vi "Hi_Tec_Control.vi"(0 "Carrier 1 Voltage":dbl(knob) min=0.0 max=5.0 scale=0.0..5.0 scale format="%.1f", 1 "Carrier 2 Voltage":dbl(knob) min=0.0 max=5.0 scale=0.0..5.0 scale format="%.1f", 2 "Trace Voltage":dbl(knob) min=0.0 max=5.0 scale=0.0..5.0 scale format="%.1f", 4 "Client Name":string) -> ()   [LabVIEW 2010]
uses:
  Anemometry/Anemometry Sub Vis/Controls/In_Range.ctl
  ADAM Client/Sub VIs/ADAM Controls/Update_scan_value.ctl
panel:
  out "Second stage":dbl[][](graph)
  out "First stage":dbl[][](graph)
  out "Increasing trace":bool
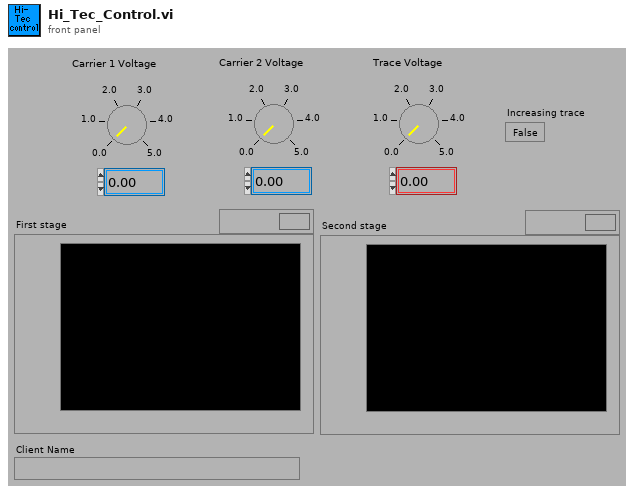
[diagram p1: front panel]
types:
  T1 = typedef "In_Range.ctl" = enum16{"%", "±", "% & ±"}
  T2 = typedef "Update_scan_value.ctl" = cluster{"Channel Name":string, "New Value":dbl}
  T3 = enum16{"Append to Global", "Read Global then Clear"}
  T4 = typedef "Ch_description_ADAM.ctl" = cluster{"Ch Name":string, "Type":T5, "Function":T6, "Ch State":T7, "Calibration type":T8, "A":dbl, "B":dbl, "C":dbl, "D":dbl, "Comments":string, "Address":T9, "String":string, "Duty":u16}
  T5 = typedef "Module_type_ADAM.ctl" = enum16{"4011", "4012", "4013", "4014", "4016", "4017", "4018", "4021", "4050", "4052", "4053", "4060", "4080", "5000", "5017", "5018", "5024", "5051", "5056", "5060", "6060", "Tracker", "WEST", "GILL", "JEM", "VICI", "Vaisala", "DRUCK", "Run VI Named:", "IR2100", "PPT", "Comparator", "VIRTUAL", "Hold Value", "Read A", "Read Ch", "Coded", "Client Info", "Web Client", "X10", "Test"}
  T6 = typedef "Function_ADAM.ctl" = enum16{"Analogue Input", "Digital Input", "Event counter", "Event rate", "Analogue Output", "Digital Output", "Relay Output"}
  T7 = typedef "Channel_State.ctl" = enum16{"On", "Off", "Always On", "Always Off"}
  T8 = typedef "Calib_type_ADAM.ctl" = enum16{"Raw", "Bx + A", "Cx^2 + Bx + A", "Dx^3 + Cx^2 + Bx + A", "In Band", "Hi-Tec Q", "Hi-Tec M_dot", "Text"}
  T9 = typedef "Address.ctl" = cluster{"Main":i32, "Ch.":i32, "Sub":i32, "Port Name":string}
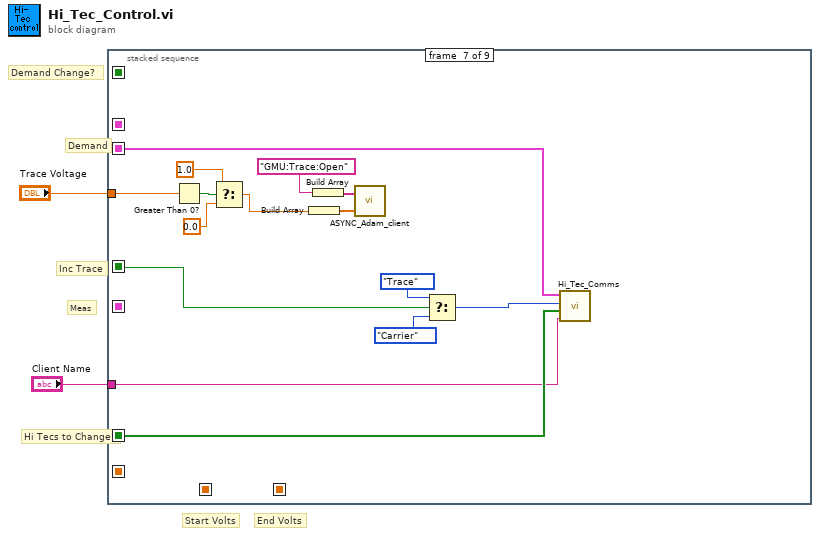
[diagram p0: block diagram]
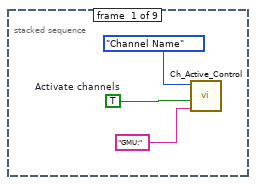
[diagram p2: hidden frame]
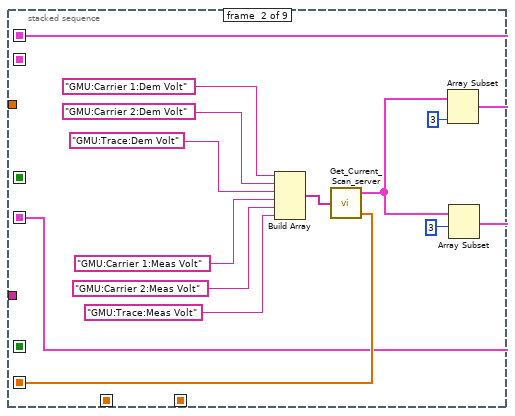
[diagram p3: hidden frame]
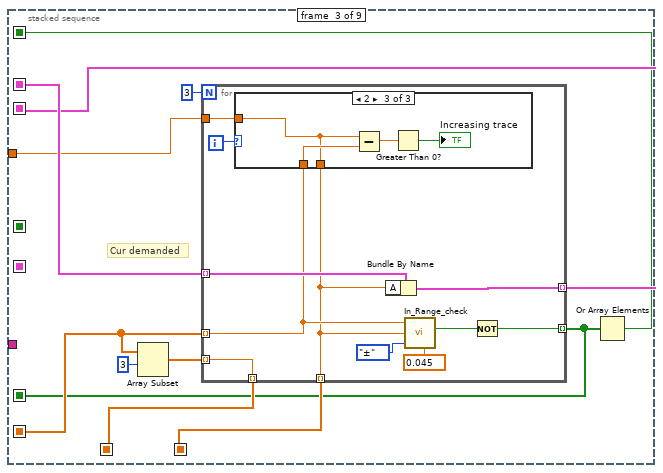
[diagram p4: hidden frame]
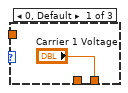
[diagram p5: hidden frame]
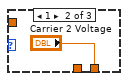
[diagram p6: hidden frame]
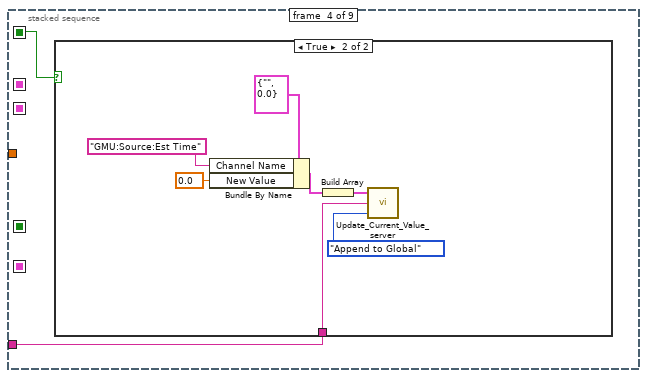
[diagram p7: hidden frame]
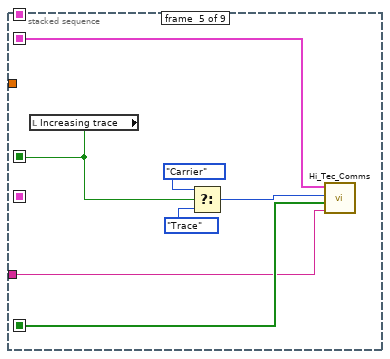
[diagram p9: hidden frame]
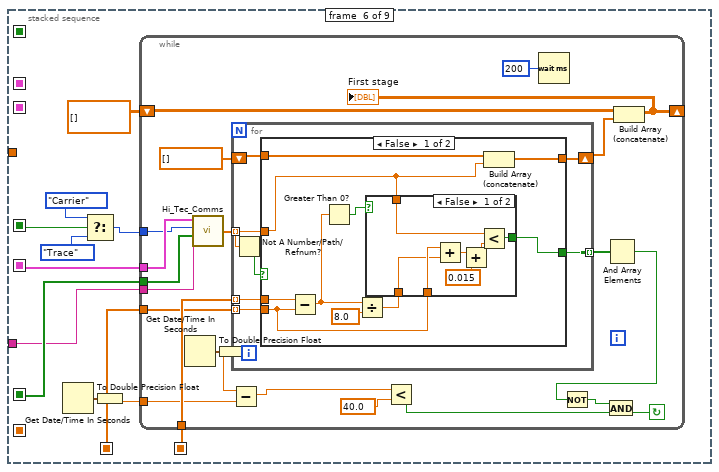
[diagram p10: hidden frame]
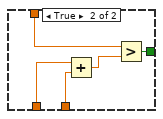
[diagram p11: hidden frame]
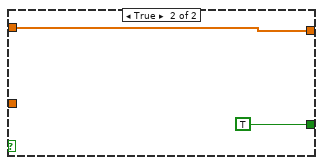
[diagram p12: hidden frame]
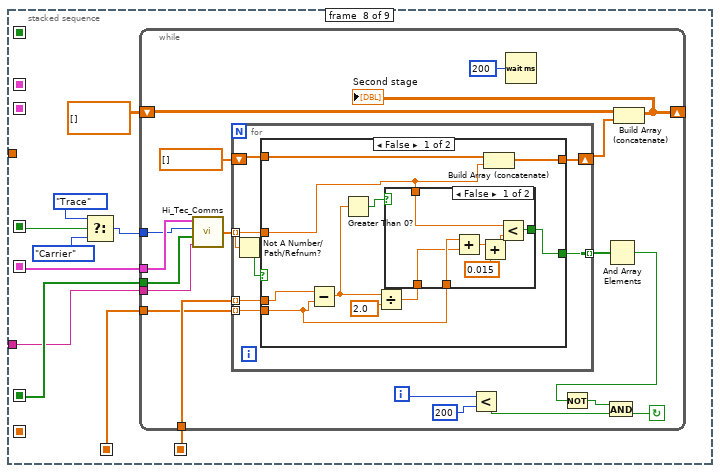
[diagram p13: hidden frame]
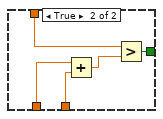
[diagram p14: hidden frame]
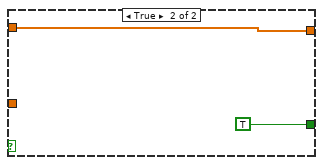
[diagram p15: hidden frame]
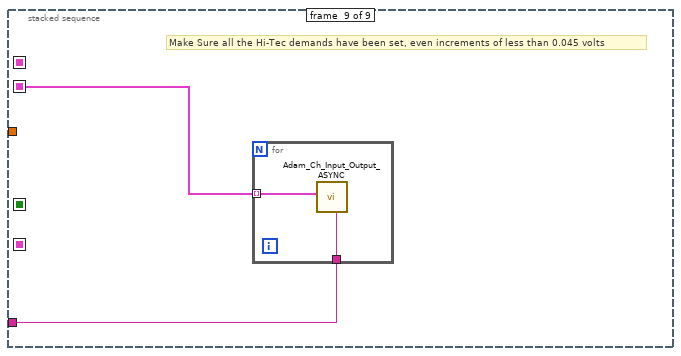
[diagram p16: hidden frame]
diagram:
  # "Demand Change?"
  # "End Volts"
  # "Start Volts"
  # "Inc Trace"
  # "Meas"
  # "Demand"
  # "Hi Tecs to Change"
  n1 = stacked-sequence {
    seq-local: [_ w12 _ _ _ _ _ _ _] -> [_ _ w29 _ _ _ _ _ _]
    seq-local: [_ w17 _ _ _ _ _ _ _] -> [_ _ w24 _ _ _ _ _ _]
    seq-local: [_ _ w21 _ _ _ _ _ _] -> [_ _ _ _ w57 w74 w137 w152 _]
    seq-local: [_ w11 _ _ _ _ _ _ _] -> [_ _ _ _ _ w70 _ w148 _]
    seq-local: [_ _ w28 _ _ _ _ _ _] -> [_ _ _ _ w58 _ w138 _ w204]
    seq-local: [_ _ _ _ w62 _ _ _ _] -> [_ _ _ _ _ w71 w142 w149 _]
    seq-local: [_ _ w27 _ _ _ _ _ _] -> [_ _ _ _ _ w67 _ w145 _]
    seq-local: [_ _ w26 _ _ _ _ _ _] -> [_ _ _ _ _ w68 _ w146 _]
    seq-local: [_ _ w20 _ _ _ _ _ _] -> [_ _ _ w47 _ _ _ _ _]
    tunnel: "Client Name" -> [_ _ _ w48 w56 w64 w136 w143 w203]
    tunnel: "Trace Voltage" -> [_ _ w19 _ _ _ w133 _ _]
    frame #0 {
      w3 = TRUE  # Activate channels
      n2 = call "Ch_Active_Control.vi"("Match"="GMU:", "Activate Channels?"=w3, "Control on"=enum16{"Channel Name", "Main Address"}."Channel Name") -> ()  [unwired: 1 in, 2 out]
    }
    frame #1 {
      n3 = Build Array("GMU:Carrier 1:Dem Volt", "GMU:Carrier 2:Dem Volt", "GMU:Trace:Dem Volt", "GMU:Carrier 1:Meas Volt", "GMU:Carrier 2:Meas Volt", "GMU:Trace:Meas Volt") -> (w18:string[])
      n4 = call "Get_Current_Scan_server.vi"("Desired Channels"=w18) -> ("Ch Description Array"=w10:T4[], "Numerical Values"=w17:dbl[])  [unwired: 1 out]
      n5 = Array Subset(array=w10, length=3 ("Array Length")) -> (w12:T4[])  [unwired: 1 in]
      n6 = Array Subset(array=w10, index=3 ("Array Length")) -> (w11:T4[])  [unwired: 1 in]
    }
    frame #2 {
      # "Cur demanded"
      n7 = Array Subset(array=w24, index=3 ("Array Index")) -> (w22:dbl[])  [unwired: 1 in]
      n8 = for {
        N: 3 -> [_]
        tunnel: w24 -> [w33] mode=indexing
        tunnel: w29 -> [w40] mode=indexing
        tunnel: [w39] -> w28 mode=indexing
        tunnel: [w36] -> w27 mode=indexing
        tunnel: [w32] -> w26 mode=indexing
        tunnel: [w37] -> w21 mode=indexing
        tunnel: w22 -> [w36] mode=indexing
        tunnel: w19 -> [w30]
        i -> [w38]
        n9 = case shown="2" w38 {
          tunnel: ["Carrier 1 Voltage" "Carrier 2 Voltage" w43] -> w32
          tunnel: w33 -> [_ _ w46]
          tunnel: w30 -> [_ _ w43]
          frame 0, Default {
          }
          frame 1 {
          }
          frame 2 {
            n10 = Subtract(x=w43, y=w46) -> (x-y=w45:dbl)
            n11 = Greater Than 0?(x=w45) -> (x > 0?=→"Increasing trace":bool)
          }
        }
        n12 = Bundle By Name(cluster=w40, "A"=w32) -> (w39:T4)
        n13 = call "In_Range_check.vi"("±"=0.045 ("%"), "Mode"=In_Range."±", "Value"=w32, "Setpoint"=w33) -> ("In Range"=w31:bool)  [unwired: 1 in, 2 out]
        n14 = Not(x=w31) -> (.not. x?=w37:bool)
      }
      n15 = Or Array Elements(Boolean array=w21) -> (logical OR=w20:bool)
    }
    frame #3 {
      n16 = case shown="True" w47 {
        tunnel: w48 -> [_ w55]
        frame False {
        }
        frame True {
          n17 = Bundle By Name(cluster=T2 {"Channel Name"="", "New Value"=0.0} ("Update Scan Value Cluster"), "Channel Name"="GMU:Source:Est Time", "New Value"=0.0 ("Bundle Element")) -> (w50:T2)
          n18 = Build Array(w50) -> (w49:T2[])
          n19 = call "Update_Current_Value_server.vi"("Mode"=T3."Append to Global", "Client HD name"=w55, "Update array in"=w49) -> ()  [unwired: 1 out]
        }
      }
    }
    frame #4 {
      n20 = local read "Increasing trace"() -> (w62:bool)
      n21 = Select(t=enum16{"Carrier", "Trace"}."Carrier" ("Type"), s=w62, f=enum16{"Carrier", "Trace"}."Trace" ("Type")) -> (s? t:f=w59:enum16{"Carrier", "Trace"})
      n22 = call "Hi_Tec_Comms.vi"("Client Name"=w56, "Hi Tec's To Change"=w57, "Type"=w59, "Ch Description Array"=w58) -> ()  [unwired: 1 out]
    }
    frame #5 {
      n23 = Get Date/Time In Seconds() -> (seconds since 1Jan1904=w63:timestamp)
      n24 = Select(t=enum16{"Carrier", "Trace"}."Carrier" ("Type"), s=w71, f=enum16{"Carrier", "Trace"}."Trace" ("Type")) -> (s? t:f=w69:enum16{"Carrier", "Trace"})
      n25 = To Double Precision Float(number=w63) -> (double precision float=w65:dbl)
      n26 = while {
        tunnel: w64 -> [w77]
        tunnel: w65 -> [w80]
        shift-left: dbl[][] [] -> [w86]
        shift-right: [w85] -> _
        tunnel: w67 -> [w93]
        tunnel: w68 -> [w94]
        tunnel: w69 -> [w95]
        tunnel: w70 -> [w96]
        tunnel: w74 -> [w87]
        stop <- w82 continue-if-true
        n27 = Get Date/Time In Seconds() -> (seconds since 1Jan1904=w76:timestamp)
        n28 = call "Hi_Tec_Comms.vi"("Client Name"=w77, "Hi Tec's To Change"=w87, "Type"=w95, "Ch Description Array"=w96) -> ("Outputs"=w92:dbl[])
        n29 = To Double Precision Float(number=w76) -> (double precision float=w81:dbl)
        n30 = Subtract(x=w81, y=w80) -> (x-y=w79:dbl)
        n31 = for {
          tunnel: w94 -> [w103] mode=indexing
          tunnel: w93 -> [w102] mode=indexing
          tunnel: w92 -> [w98] mode=indexing
          tunnel: [w101] -> w91 mode=indexing
          shift-right: [w99] -> w88
          shift-left: dbl[] [] -> [w100]
          n32 = Not A Number/Path/Refnum?(number/path/refnum=w98) -> (NaN/Path/Refnum?=w97:bool)
          n33 = case shown="False" w97 {
            tunnel: w103 -> [w110 _]
            tunnel: w102 -> [w106 _]
            tunnel: w98 -> [w105 _]
            tunnel: [w104 TRUE] -> w101
            tunnel: w100 -> [w109 w126]
            tunnel: [w108 w126] -> w99
            frame False {
              n34 = Subtract(x=w110, y=w106) -> (x-y=w112:dbl)
              n35 = Greater Than 0?(x=w112) -> (x > 0?=w111:bool)
              n36 = Divide(x=w112, y=8.0) -> (x/y=w107:dbl)
              n37 = case shown="False" w111 {
                tunnel: w107 -> [w119 w125]
                tunnel: w106 -> [w120 w124]
                tunnel: w105 -> [w118 w122]
                tunnel: [w117 w121] -> w104
                frame False {
                  n38 = Add(x=w120, y=w119) -> (x+y=w116:dbl)
                  n39 = Add(x=w116, y=0.015 ("x")) -> (x+y=w115:dbl)
                  n40 = Less?(x=w118, y=w115) -> (x < y?=w117:bool)
                }
                frame True {
                  n41 = Add(x=w125, y=w124) -> (x+y=w123:dbl)
                  n42 = Greater?(x=w122, y=w123) -> (0:w121:bool)
                }
              }
              n43 = Build Array (concatenate)(w109, w105) -> (w108:dbl[])
            }
            frame True {
            }
          }
        }
        n44 = Less?(x=w79, y=40.0) -> (x < y?=w84:bool)
        n45 = Wait (ms)(milliseconds to wait=u32 200) -> ()  [unwired: 1 out]
        n46 = And Array Elements(Boolean array=w91) -> (logical AND=w90:bool)
        n47 = Not(x=w90) -> (.not. x?=w83:bool)
        n48 = And(x=w83, y=w84) -> (x .and. y?=w82:bool)
        n49 = Build Array (concatenate)(w86, w88) -> (w85:dbl[][])
        "First stage" <- w85
      }
    }
    frame #6 {
      n50 = Greater Than 0?(x=w133) -> (x > 0?=w132:bool)
      n51 = Select(t=1.0, s=w132, f=0.0) -> (s? t:f=w129:dbl)
      n52 = Build Array(w129) -> (w134:dbl[])
      n53 = Build Array("GMU:Trace:Open") -> (w135:string[])
      n54 = call "ASYNC_Adam_client.vi"("Values"=w134, "Channel Names"=w135) -> ()  [unwired: 2 out]
      n55 = Select(t=enum16{"Carrier", "Trace"}."Trace" ("Type"), s=w142, f=enum16{"Carrier", "Trace"}."Carrier" ("Type")) -> (s? t:f=w139:enum16{"Carrier", "Trace"})
      n56 = call "Hi_Tec_Comms.vi"("Client Name"=w136, "Hi Tec's To Change"=w137, "Type"=w139, "Ch Description Array"=w138) -> ()  [unwired: 1 out]
    }
    frame #7 {
      n57 = Select(t=enum16{"Carrier", "Trace"}."Trace" ("Type"), s=w149, f=enum16{"Carrier", "Trace"}."Carrier" ("Type")) -> (s? t:f=w147:enum16{"Carrier", "Trace"})
      n58 = while {
        tunnel: w143 -> [w154]
        shift-left: dbl[][] [] -> [w161]
        shift-right: [w155] -> _
        tunnel: w145 -> [w168]
        tunnel: w146 -> [w169]
        tunnel: w147 -> [w170]
        tunnel: w148 -> [w171]
        tunnel: w152 -> [w162]
        i -> [w157]
        stop <- w156 continue-if-true
        n59 = call "Hi_Tec_Comms.vi"("Client Name"=w154, "Hi Tec's To Change"=w162, "Type"=w170, "Ch Description Array"=w171) -> ("Outputs"=w167:dbl[])
        n60 = for {
          tunnel: w169 -> [w178] mode=indexing
          tunnel: w168 -> [w177] mode=indexing
          tunnel: w167 -> [w173] mode=indexing
          tunnel: [w176] -> w166 mode=indexing
          shift-right: [w174] -> w163
          shift-left: dbl[] [] -> [w175]
          n61 = Not A Number/Path/Refnum?(number/path/refnum=w173) -> (NaN/Path/Refnum?=w172:bool)
          n62 = case shown="False" w172 {
            tunnel: w178 -> [w182 _]
            tunnel: w177 -> [w181 _]
            tunnel: w173 -> [w180 _]
            tunnel: [w179 TRUE] -> w176
            tunnel: w175 -> [w188 w201]
            tunnel: [w187 w201] -> w174
            frame False {
              n63 = Subtract(x=w182, y=w181) -> (x-y=w185:dbl)
              n64 = Greater Than 0?(x=w185) -> (x > 0?=w184:bool)
              n65 = Divide(x=w185, y=2.0) -> (x/y=w183:dbl)
              n66 = case shown="False" w184 {
                tunnel: w183 -> [w194 w200]
                tunnel: w181 -> [w195 w199]
                tunnel: w180 -> [w193 w197]
                tunnel: [w192 w196] -> w179
                frame False {
                  n67 = Add(x=w195, y=w194) -> (x+y=w191:dbl)
                  n68 = Add(x=w191, y=0.015 ("x")) -> (x+y=w190:dbl)
                  n69 = Less?(x=w193, y=w190) -> (x < y?=w192:bool)
                }
                frame True {
                  n70 = Add(x=w200, y=w199) -> (x+y=w198:dbl)
                  n71 = Greater?(x=w197, y=w198) -> (0:w196:bool)
                }
              }
              n72 = Build Array (concatenate)(w188, w180) -> (w187:dbl[])
            }
            frame True {
            }
          }
        }
        n73 = Less?(x=w157, y=200) -> (x < y?=w159:bool)
        n74 = Wait (ms)(milliseconds to wait=u32 200) -> ()  [unwired: 1 out]
        n75 = And Array Elements(Boolean array=w166) -> (logical AND=w165:bool)
        n76 = Not(x=w165) -> (.not. x?=w158:bool)
        n77 = And(x=w158, y=w159) -> (x .and. y?=w156:bool)
        n78 = Build Array (concatenate)(w161, w163) -> (w155:dbl[][])
        "Second stage" <- w155
      }
    }
    frame #8 {
      # "Make Sure all the Hi-Tec demands have been set, even increments of less than 0.045 volts"
      n79 = for {
        tunnel: w204 -> [w206] mode=indexing
        tunnel: w203 -> [w205]
        n80 = call "Adam_Ch_Input_Output_ASYNC.vi"("Client Name"=w205, "Ch Discription"=w206) -> ()  [unwired: 5 in, 5 out]
      }
    }
  }
